vi "refRidders Zero Inner Part.vi"(0 "start/end/f(x)":T2 {"end" format="%.2f"; "start" format="%.2f"; "y value copy" format="%.2f"; "y value" format="%.2f"}, 1 "Variant":variant, 2 "function refnum":T1, 3 "level":dbl, 4 "accuracy":dbl format="%.2f", 5 "case":bool) -> (6 "y value":dbl format="%.2f", 7 "end":dbl format="%.2f", 8 "error":i32)   [LabVIEW 2014, in "NI_Gmath.lvlib"]
uses:
  NI_Gmath.lvlib
  functionRefnum.ctl
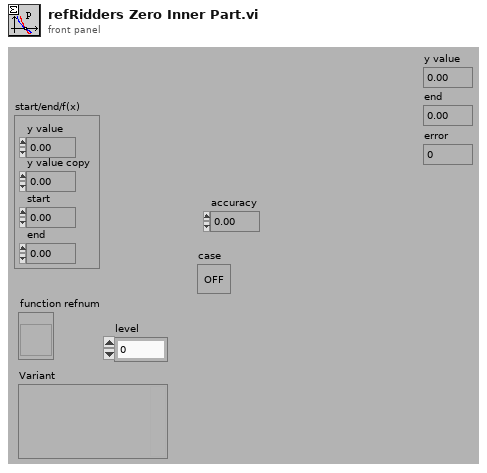
[diagram p1: front panel]
types:
  T1 = typedef "NI_Gmath.lvlib/functionRefnum.ctl" = refnum<vi>
  T2 = cluster{"y value":dbl, "y value copy":dbl, "start":dbl, "end":dbl}
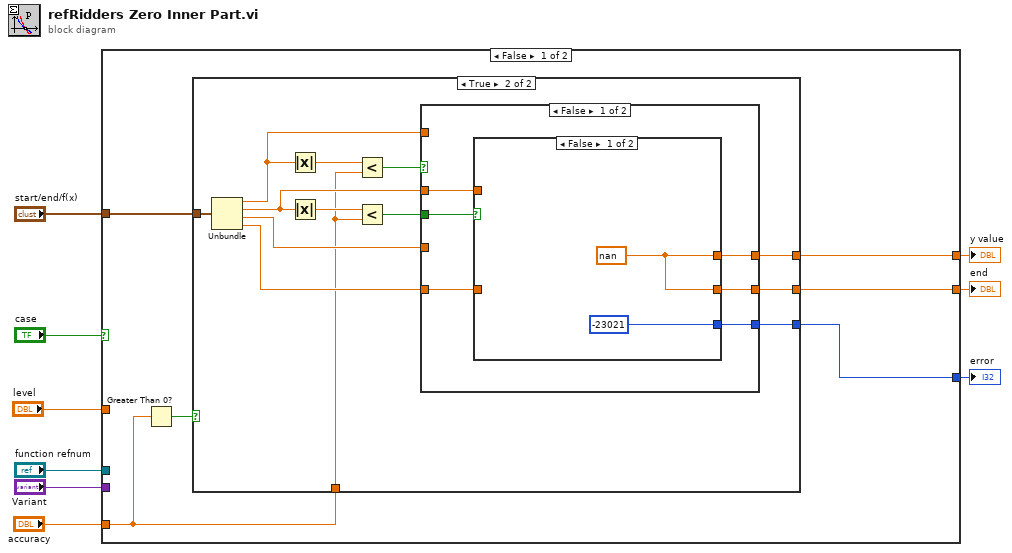
[diagram p0: block diagram]
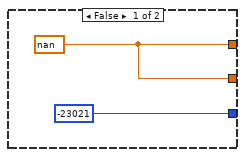
[diagram p2: hidden frame]
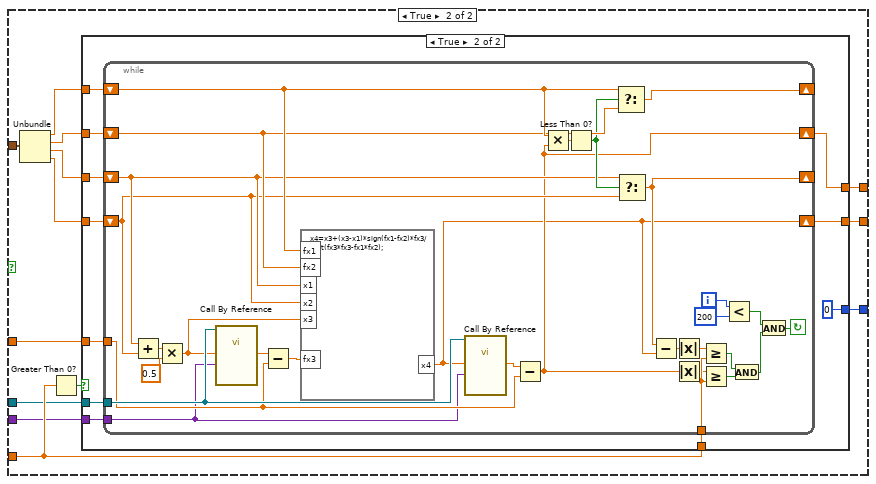
[diagram p5: hidden frame]
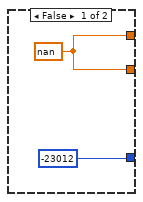
[diagram p6: hidden frame]
diagram:
  n1 = case shown="False" "case" {
    tunnel: [w12 w54] -> w5
    tunnel: "accuracy" -> [w11 w51]
    tunnel: [w13 w53] -> w7
    tunnel: [w14 w52] -> w8
    tunnel: "start/end/f(x)" -> [w15 w50]
    tunnel: "function refnum" -> [_ w45]
    tunnel: "Variant" -> [_ w44]
    tunnel: "level" -> [_ w43]
    frame False {
      n2 = Greater Than 0?(x=w11) -> (x > 0?=w10:bool)
      n3 = case shown="True" w10 {
        tunnel: w15 -> [_ w22]
        tunnel: [w17 w21] -> w14
        tunnel: [w17 w20] -> w13
        tunnel: [-23021 w19] -> w12
        tunnel: w11 -> [_ w18]
        frame False {
          w17 = nan ("y value copy")
        }
        frame True {
          n4 = Unbundle(w22) -> ("y value"=w27:dbl, "y value copy"=w24:dbl, "start"=w26:dbl, "end"=w25:dbl)
          n5 = Absolute Value(x=w27) -> (abs(x)=w30:dbl)
          n6 = Absolute Value(x=w24) -> (abs(x)=w29:dbl)
          n7 = Less?(x=w30, y=w18) -> (x < y?=w28:bool)
          n8 = Less?(x=w29, y=w18) -> (x < y?=w23:bool)
          n9 = case shown="False" w28 {
            tunnel: w27 -> [_ w42]
            tunnel: w26 -> [_ w41]
            tunnel: w25 -> [w32 _]
            tunnel: w24 -> [w34 _]
            tunnel: [w35 w42] -> w21
            tunnel: [w33 w41] -> w20
            tunnel: w23 -> [w36 _]
            tunnel: [w31 _] -> w19
            frame False {
              n10 = case shown="False" w36 {
                tunnel: [w38 w40] -> w35
                tunnel: w34 -> [_ w40]
                tunnel: [w38 w39] -> w33
                tunnel: w32 -> [_ w39]
                tunnel: [-23021 _] -> w31
                frame False {
                  w38 = nan ("y value copy")
                }
                frame True {
                }
              }
            }
            frame True {
            }
          }
        }
      }
    }
    frame True {
      n11 = Unbundle(w50) -> ("y value"=w46:dbl, "y value copy"=w47:dbl, "start"=w48:dbl, "end"=w49:dbl)
      n12 = Greater Than 0?(x=w51) -> (x > 0?=w55:bool)
      n13 = case shown="True" w55 {
        tunnel: w51 -> [_ w68]
        tunnel: w46 -> [_ w67]
        tunnel: w47 -> [_ w66]
        tunnel: w48 -> [_ w65]
        tunnel: w49 -> [_ w64]
        tunnel: [-23012 0] -> w54
        tunnel: [w56 w62] -> w53
        tunnel: [w56 w61] -> w52
        tunnel: w45 -> [_ w60]
        tunnel: w44 -> [_ w59]
        tunnel: w43 -> [_ w58]
        frame False {
          w56 = nan
        }
        frame True {
          n14 = while {
            tunnel: w68 -> [w97]
            shift-left: w66 -> [w81]
            shift-right: [w74] -> w61
            shift-left: w67 -> [w83]
            shift-right: [w82] -> _
            shift-left: w64 -> [w77]
            shift-right: [w69] -> w62
            shift-left: w65 -> [w78]
            shift-right: [w79] -> _
            tunnel: w60 -> [w98]
            tunnel: w59 -> [w70]
            tunnel: w58 -> [w75]
            i -> [w90]
            stop <- w87 continue-if-true
            n15 = Add(x=w78, y=w77) -> (x+y=w95:dbl)
            n16 = Multiply(x=w95, y=0.5) -> (x*y=w72:dbl)
            n17 = call-by-ref "?"(reference=w98, "Variant"=w70, "x"=w72) -> ("f(x)"=w73:dbl)  [unwired: 4 in, 2 out]
            n18 = Subtract(x=w73, y=w75) -> (x-y=w76:dbl)
            n19 = formula code="x4=x3+(x3-x1)*sign(fx1-fx2)*fx3/sqrt(fx3*fx3-fx1*fx2);"("fx1"=w83, "fx2"=w81, "fx3"=w76, "x1"=w78, "x2"=w77, "x3"=w72) -> ("x4"=w69:dbl)
            n20 = call-by-ref "?"(reference=w98, "Variant"=w70, "x"=w69) -> ("f(x)"=w71:dbl)  [unwired: 4 in, 2 out]
            n21 = Subtract(x=w71, y=w75) -> (x-y=w74:dbl)
            n22 = Multiply(x=w83, y=w74) -> (x*y=w94:dbl)
            n23 = Less Than 0?(x=w94) -> (x < 0?=w80:bool)
            n24 = Select(t=w83, s=w80, f=w81) -> (s? t:f=w82:dbl)
            n25 = Select(t=w78, s=w80, f=w77) -> (s? t:f=w79:dbl)
            n26 = Subtract(x=w79, y=w69) -> (x-y=w92:dbl)
            n27 = Absolute Value(x=w92) -> (abs(x)=w93:dbl)
            n28 = Absolute Value(x=w74) -> (abs(x)=w91:dbl)
            n29 = Greater Or Equal?(x=w93, y=w97) -> (x >= y?=w84:bool)
            n30 = Greater Or Equal?(x=w91, y=w97) -> (x >= y?=w85:bool)
            n31 = Less?(x=w90, y=200) -> (x < y?=w88:bool)
            n32 = And(x=w84, y=w85) -> (x .and. y?=w86:bool)
            n33 = And(x=w88, y=w86) -> (x .and. y?=w87:bool)
          }
        }
      }
    }
  }
  "y value" <- w8
  "end" <- w7
  "error" <- w5
